vi "extract_openai_embeddings.vi"(10 "body":string, 11 "headers":string) -> (0 "error out":errorcluster, 3 "vector response":refnum<class "message_vectors.lvclass">)   [LabVIEW 2020, in "llm_openai_embedding.lvclass"]
uses:
  llm_openai_embedding.lvclass
  message_vectors/message_vectors.lvclass
  message_vectors/embedding.ctl
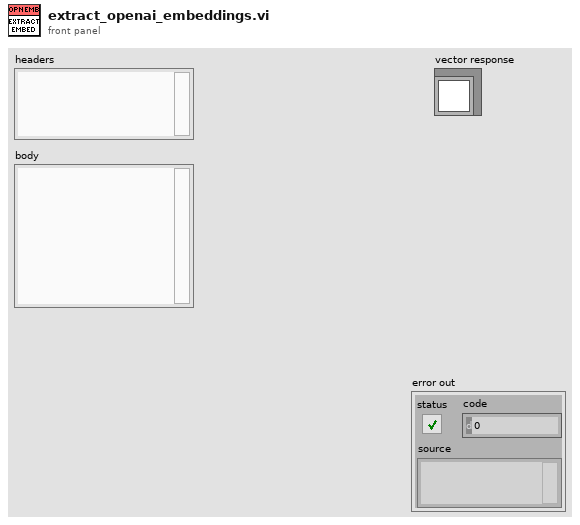
[diagram p1: front panel]
types:
  T1 = typedef "message_vectors.lvclass/embedding.ctl" = cluster{"index":u32, "Vectors":dbl[]}
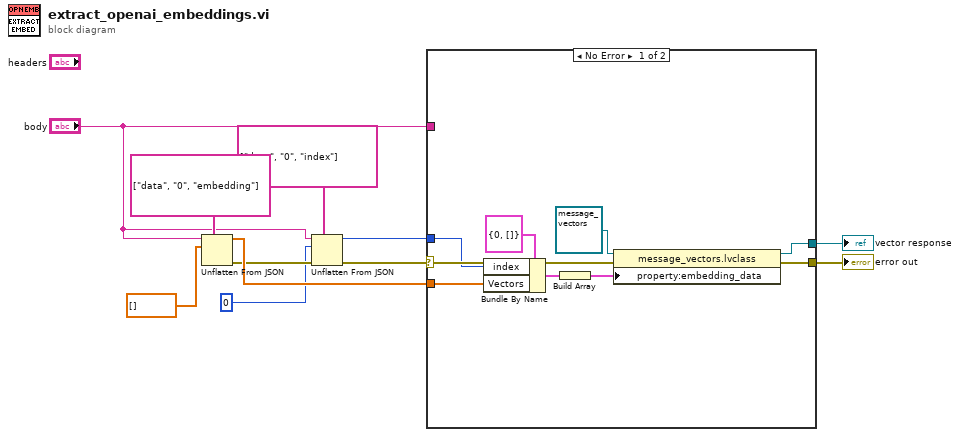
[diagram p0: block diagram]
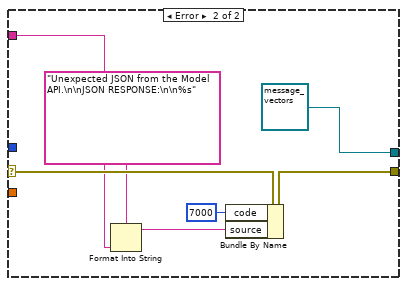
[diagram p2: hidden frame]
diagram:
  n1 = Unflatten From JSON(path=string[] ["data", "0", "embedding"], JSON string="body", type and defaults=dbl[] []) -> (value=w9:dbl[], error out=w6:errorcluster)  [unwired: 4 in]
  n2 = Unflatten From JSON(path=string[] ["data", "0", "index"], JSON string="body", type and defaults=u32 0, error in (no error)=w6) -> (value=w1:u32, error out=w5:errorcluster)  [unwired: 3 in]
  n3 = case shown="No Error" w5 {
    selector: w5 -> [w15 w26]
    tunnel: w9 -> [w18 _]
    tunnel: [w14 refnum<class "message_vectors.lvclass"> refnum ("message_vectors.lvclass")] -> w8
    tunnel: [w13 w21] -> w7
    tunnel: "body" -> [_ w25]
    tunnel: w1 -> [w12 _]
    frame No Error {
      n4 = Bundle By Name(cluster=T1 {"index"=0, "Vectors"=[]} ("embedding"), "index"=w12, "Vectors"=w18) -> (w17:T1)
      n5 = Build Array(w17) -> (w16:T1[])
      n6 = property class="message_vectors.lvclass"(reference=refnum<class "message_vectors.lvclass"> refnum ("message_vectors.lvclass"), error in=w15, "property:embedding_data"=w16) -> (reference out=w14:refnum<class "message_vectors.lvclass">, error out=w13:errorcluster)
    }
    frame Error {
      n7 = Format Into String(format string="Unexpected JSON from the Model API.\n\nJSON RESPONSE:\n\n%s", w25) -> (resulting string=w23:string)  [unwired: 2 in, 1 out]
      n8 = Bundle By Name(cluster=w26, "code"=7000, "source"=w23) -> (w21:errorcluster)
    }
  }
  "vector response" <- w8
  "error out" <- w7
